vi "initialiseCam.vi"(8 "error in (no error)":errorcluster, 9 "Control name":string, 10 "viPath":string="Hal\\Channels\\Camera\\Camera\\Pixelfly\\initialise.vi", 11 "NetworkCamera in":refnum<class "NetworkCamera.lvclass">) -> (0 "error out":errorcluster, 3 "NetworkCamera out":refnum<class "NetworkCamera.lvclass">)   [LabVIEW 2009, in "Hardware.lvlib" / "HWControllers.lvlib" / "NetworkCamera.lvclass"]
uses:
  NetworkCamera.lvclass
  Channels/Camera/Camera/Camera.lvclass
  NetworkCamera.lvclass/NetworkCamera.ctl
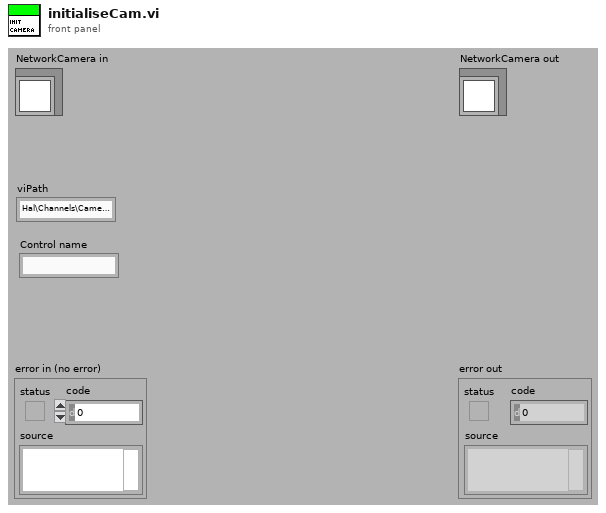
[diagram p1: front panel]
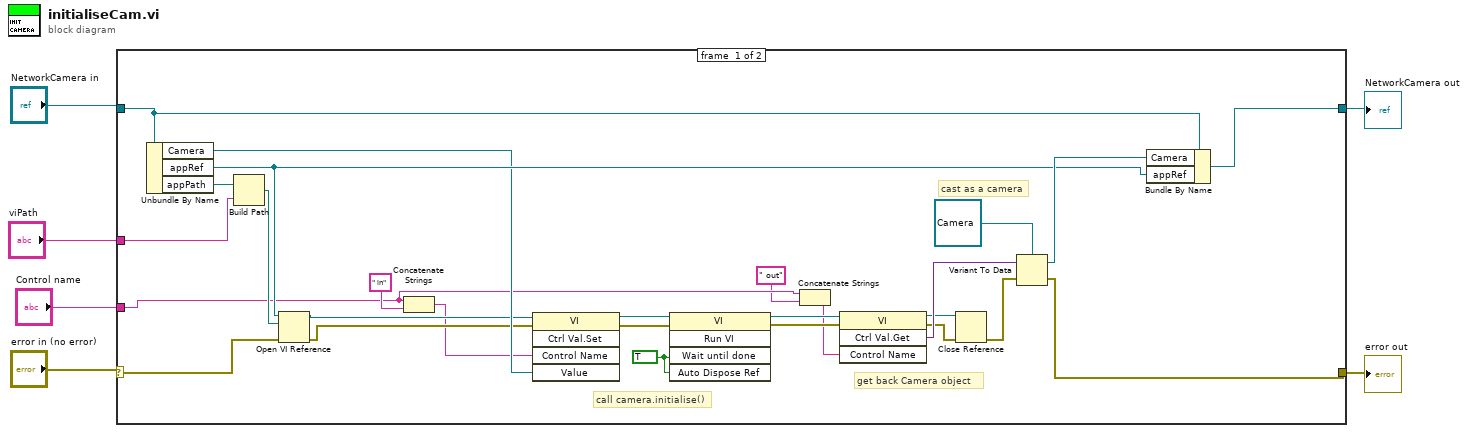
[diagram p0: block diagram]
diagram:
  n1 = case shown="No Error" "error in (no error)" {
    selector: "error in (no error)" -> [w16 w35]
    tunnel: [w22 w35] -> w3
    tunnel: [w20 w34] -> w4
    tunnel: "NetworkCamera in" -> [w19 w34]
    tunnel: "viPath" -> [w12 _]
    tunnel: "Control name" -> [w9 _]
    frame #0 {
      w30 = TRUE
      # "get back Camera object"
      # "call camera.initialise()"
      # "cast as a camera"
      n2 = Unbundle By Name(w19) -> ("Camera"=w15:refnum<class "Camera.lvclass">, "appRef"=w17:refnum<vi>, "appPath"=w18:path)
      n3 = Build Path(base path=w18, name or relative path=w12) -> (appended path=w33:path)
      n4 = Open VI Reference(application reference (local)=w17, vi path=w33, error in (no error)=w16) -> (vi reference=w14:refnum<vi>, error out=w13:errorcluster)  [unwired: 3 in]
      n5 = Concatenate Strings(w9, " in") -> (w10:string)
      n6 = invoke class="VI" method="Ctrl Val.Set"(reference=w14, error in=w13, "Control Name"=w10, "Value"=w15) -> (reference out=w32:refnum<vi>, error out=w31:errorcluster)  [unwired: 1 in, 3 out]
      n7 = invoke class="VI" method="Run VI"(reference=w32, error in=w31, "Wait until done"=w30, "Auto Dispose Ref"=w30) -> (reference out=w29:refnum<vi>, error out=w28:errorcluster)  [unwired: 1 in, 3 out]
      n8 = Concatenate Strings(w9, " out") -> (w7:string)
      n9 = invoke class="VI" method="Ctrl Val.Get"(reference=w29, error in=w28, "Control Name"=w7) -> (reference out=w24:refnum<vi>, error out=w25:errorcluster, "Get Control Value Variant"=w26:variant)  [unwired: 1 in, 1 out]
      n10 = Close Reference(reference=w24, error in (no error)=w25) -> (error out=w23:errorcluster)
      n11 = Variant To Data(error in=w23, Variant=w26, type=refnum<class "Camera.lvclass"> refnum ("Camera out")) -> (error out=w22:errorcluster, data=w21:refnum<class "Camera.lvclass">)
      n12 = Bundle By Name(cluster=w19, "Camera"=w21, "appRef"=w17) -> (w20:refnum<class "NetworkCamera.lvclass">)
    }
    frame #1 {
    }
  }
  "error out" <- w3
  "NetworkCamera out" <- w4
